vi "UpdateStatusForInvalidEstimation.vi"(8 "error in":errorcluster, 9 "invalid estimation?":bool=TRUE, 11 "data map":T1) -> (0 "error out":errorcluster, 3 "data map out":T1)   [LabVIEW 2017, in "McsaAnalysisFunctions.lvlib"]
uses:
  <vilib>/addons/InsightCM/Utilities/Analysis/MCSA/McsaAnalysisFunctions.lvlib
  <vilib>/addons/PointValueMap/controls/PointMap.ctl
  <vilib>/addons/PointValueMap/PointValueMap.lvlib
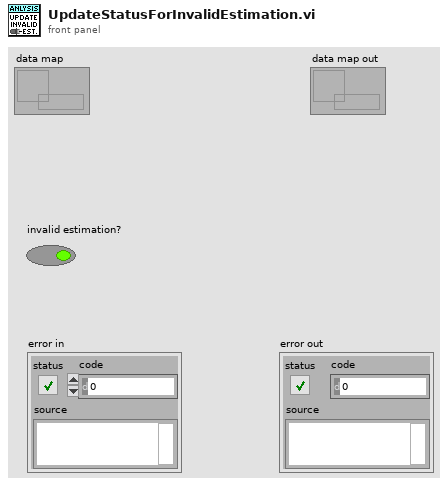
[diagram p1: front panel]
types:
  T1 = typedef "PointValueMap.lvlib/PointMap.ctl" = refnum<data-value>
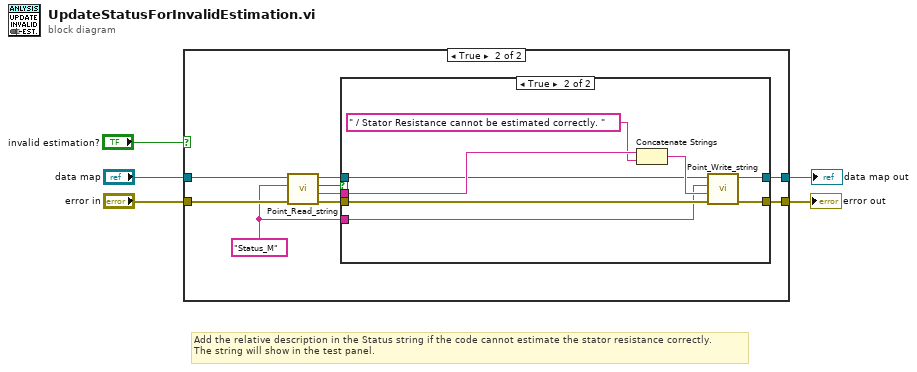
[diagram p0: block diagram]
diagram:
  # "Add the relative description in the Status string if the code cannot estimate the stator resistance correctly.\nThe string will show in the test panel."
  n1 = case shown="True" "invalid estimation?" {
    tunnel: "error in" -> [w7 w16]
    tunnel: "data map" -> [w6 w15]
    tunnel: [w7 w12] -> w3
    tunnel: [w6 w8] -> w1
    frame False {
    }
    frame True {
      w9 = "Status_M" ("string")
      n2 = call <vilib>:"Point_Read_string.vi"("Error In"=w16, "Tag"=w9, "Map"=w15) -> ("Error Out"=w11:errorcluster, "Value"=w13:string, "Found?"=w14:bool, "Map Out"=w10:T1)  [unwired: 3 in, 2 out]
      n3 = case shown="True" w14 {
        tunnel: w13 -> [_ w26]
        tunnel: [w18 w23] -> w12
        tunnel: w11 -> [w18 w24]
        tunnel: w10 -> [w17 w21]
        tunnel: w9 -> [_ w20]
        tunnel: [w17 w19] -> w8
        frame False {
        }
        frame True {
          n4 = Concatenate Strings(w26, " / Stator Resistance cannot be estimated correctly. " ("string")) -> (w22:string)
          n5 = call <vilib>:"Point_Write_string.vi"("Error In"=w24, "Value"=w22, "Tag"=w20, "Map"=w21) -> ("Error Out"=w23:errorcluster, "Map Out"=w19:T1)  [unwired: 6 in]
        }
      }
    }
  }
  "error out" <- w3
  "data map out" <- w1
